vi "Open Hardware.vi"(8 "error in (no error)":errorcluster, 11 "VISA Refnum in":refnum<visa-resource-name>) -> (0 "error out":errorcluster, 3 "VISA Refnum out":refnum<visa-resource-name>)   [LabVIEW 2019]
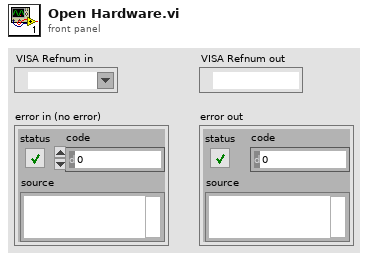
[diagram p1: front panel]
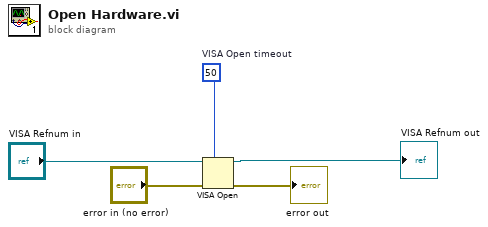
[diagram p0: block diagram]
diagram:
  w1 = u32 50  # VISA Open timeout
  n1 = VISA Open(timeout (0)=w1, error in (no error)="error in (no error)", VISA resource name="VISA Refnum in") -> (VISA resource name=→"VISA Refnum out":refnum<visa-resource-name>, error out=→"error out":errorcluster)  [unwired: 2 in]
